vi "Select Keywords Method.vi"(0 "Display State In":T1, 9 "Container State":T2, 11 "error in (no error)":errorcluster) -> (4 "Display State Out":T1, 15 "error out":errorcluster)   [LabVIEW 2012, in "Intellisense Xcontrol.xctl"]
uses:
  Intellisense Xcontrol.xctl
  <vilib>/_xctls/Container State.ctl
  State 1.ctl
  <vilib>/_xctls/XControlSupport.lvlib
panel:
  # "Add Controls & Indicators that form the parameters of the method here. Hook them to the connector pane. Do not delete the controls & indicators that are already hooked to the connector pane.\n \nTo setup the parameters  for this method, right click on this item in the Project Tree & select \"Configure Method...\"."
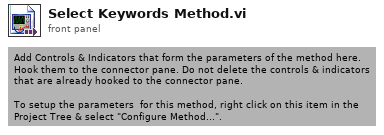
[diagram p1: front panel]
types:
  T1 = typedef "Intellisense Xcontrol.xctl/State 1.ctl" = cluster{"Keyword Array":string[], "Auto-Complete On/Off":bool, "Delimiter":string}
  T2 = typedef "XControlSupport.lvlib/Container State.ctl" = cluster{"Indicator?":bool, "Run Mode?":bool, " Refnum":refnum<vi>}
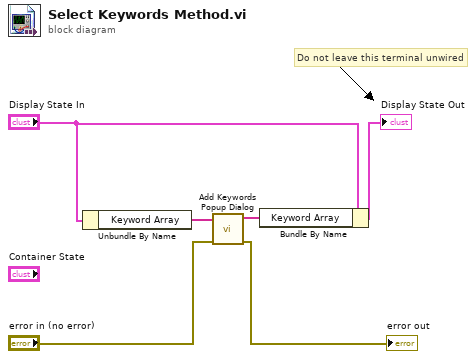
[diagram p0: block diagram]
diagram:
  # "Do not leave this terminal unwired"
  n1 = Unbundle By Name("Display State In") -> ("Keyword Array"=w5:string[])
  n2 = call "Add Keywords Popup Dialog.vi"("error in (no error)"="error in (no error)", "Keywords In"=w5) -> ("error out"=→"error out":errorcluster, "Keywords Out"=w4:string[])  [unwired: 8 in]
  n3 = Bundle By Name(cluster="Display State In", "Keyword Array"=w4) -> (→"Display State Out":T1)
